vi "editscenario handle delete scenario.vi"(6 "User Information":T2, 8 "error in (no error)":errorcluster, 10 "scenarioId (\"\")":string, 11 "Connection Refnum":T1) -> (0 "error out":errorcluster, 3 "Connection Refnum":T1)   [LabVIEW 2011]
uses:
  server/database/Users/User Record.ctl
  SI.LIB/ODBC/SQL Controls/Connection Refnum.ctl
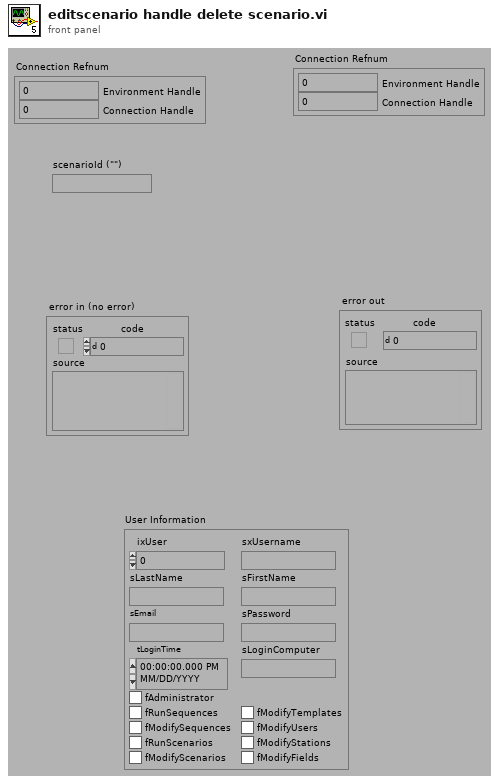
[diagram p1: front panel]
types:
  T1 = typedef "Connection Refnum.ctl" = cluster{"Environment Handle":i32, "Connection Handle":i32}
  T2 = typedef "User Record.ctl" = cluster{"ixUser":i32, "sxUsername":string, "sLastName":string, "sFirstName":string, "sEmail":string, "sPassword":string, "tLoginTime":timestamp, "sLoginComputer":string, "fAdministrator":bool, "fRunSequences":bool, "fModifySequences":bool, "fRunScenarios":bool, "fModifyScenarios":bool, "fModifyTemplates":bool, "fModifyUsers":bool, "fModifyStations":bool, "fModifyFields":bool}
  T3 = typedef "Scenario Record.ctl" = cluster{"ixScenario":i32, "tCreated":timestamp, "tModified":timestamp, "sxUsername":string, "sModifiedBy":string, "sxScenarioId":string, "sDescription":string, "sLogic":string, "sResultFieldsCSV":string, "sTemplatesCSV":string, "fAutoRunReports":bool, "fSortByTemplates":bool, "fCombinePDF":bool, "Conditions":T4[]}
  T4 = typedef "Condition Record.ctl" = cluster{"iConditionIndex":i32, "sxFieldId":string, "nOperator":T5, "sMatchValue":string}
  T5 = typedef "Condition Operators.ctl" = enum16{"equal (=)", "not equal (\\u2260)", "less than (<)", "less than or equal (\\u2264)", "greater than (>)", "greater than or equal (\\u2265)", "contains", "does not contain"}
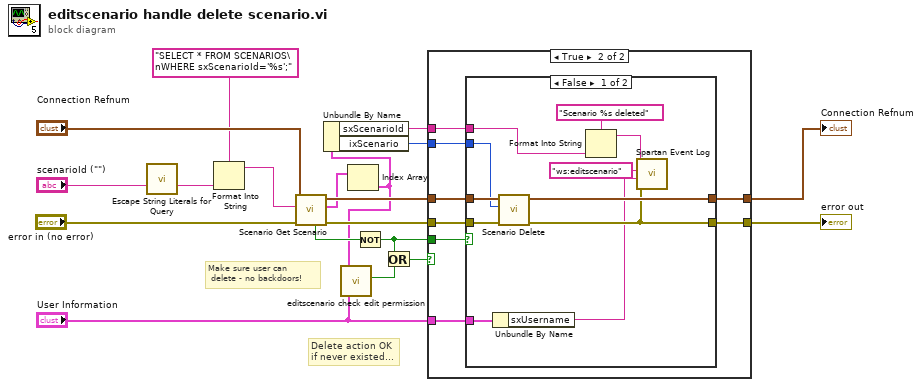
[diagram p0: block diagram]
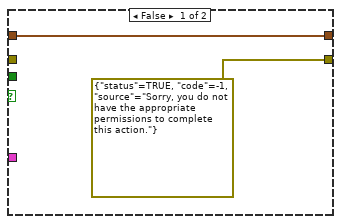
[diagram p2: hidden frame]
diagram:
  # "Delete action OK\nif never existed..."
  # "Make sure user can\n delete - no backdoors!"
  n1 = call "Escape String Literals for Query.vi"("String"="scenarioId (\"\")") -> ("escaped String"=w5:string)  [unwired: 1 in, 13 out]
  n2 = Format Into String(format string="SELECT * FROM SCENARIOS\nWHERE sxScenarioId='%s';", w5) -> (resulting string=w6:string)  [unwired: 2 in, 1 out]
  n3 = call "Scenario Get Scenario.vi"("error in (no error)"="error in (no error)", "Query"=w6, "Connection Refnum"="Connection Refnum") -> ("error out"=w17:errorcluster, "Scenarios"=w4:T3[], "Connection Refnum"=w15:T1, "Data Present?"=w12:bool)  [unwired: 5 out]
  n4 = Index Array(array=w4) -> (element=w1:T3)  [unwired: 1 in]
  n5 = Unbundle By Name(w1) -> ("sxScenarioId"=w2:string, "ixScenario"=w3:i32)
  n6 = call "editscenario check edit permission.vi"("User Information"="User Information", "Scenario Record"=w1) -> ("Okay to Edit?"=w11:bool)  [unwired: 5 out]
  n7 = Not(x=w12) -> (.not. x?=w9:bool)
  n8 = Or(x=w9, y=w11) -> (x .or. y?=w10:bool)
  n9 = case shown="True" w10 {
    tunnel: [w21 w29] -> w19
    tunnel: [errorcluster {"status"=TRUE, "code"=-1, "source"="Sorry, you do not have the appropriate permissions to complete this action."} ("error out") w28] -> w18
    tunnel: w17 -> [_ w27]
    tunnel: w15 -> [w21 w26]
    tunnel: "User Information" -> [_ w24]
    tunnel: w3 -> [_ w25]
    tunnel: w9 -> [_ w23]
    tunnel: w2 -> [_ w22]
    frame False {
    }
    frame True {
      n10 = case shown="False" w23 {
        tunnel: [w37 w42] -> w29
        tunnel: [w36 w41] -> w28
        tunnel: w27 -> [w35 w41]
        tunnel: w26 -> [w34 w42]
        tunnel: w25 -> [w33 _]
        tunnel: w24 -> [w32 _]
        tunnel: w22 -> [w30 _]
        frame False {
          n11 = Unbundle By Name(w32) -> ("sxUsername"=w31:string)
          n12 = call "Scenario Delete.vi"("error in (no error)"=w35, "ixScenario (0)"=w33, "Connection Refnum"=w34) -> ("error out"=w36:errorcluster, "Connection Refnum"=w37:T1)  [unwired: 7 out]
          n13 = Format Into String(format string="Scenario %s deleted" ("message (\"\")"), w30) -> (resulting string=w39:string)  [unwired: 2 in, 1 out]
          n14 = call "Spartan Event Log.vi"("error in (no error)"=w36, "username (\"\")"=w31, "module (\"\")"="ws:editscenario", "message (\"\")"=w39) -> ()  [unwired: 4 in, 1 out]
        }
        frame True {
          # "No record to delete - move on..."
        }
      }
    }
  }
  "error out" <- w18
  "Connection Refnum" <- w19
